vi "Prueba_comandos.vi"() -> ()   [LabVIEW 2010]
uses:
  <vilib>/Instr/_visa.llb/VISA Configure Serial Port (Instr).vi
panel:
  out "Comando leido":string
  in  "Leer":bool
  in  "Comando a escribir":string="WTt1 000000000"
  in  "Escribir":bool
  in  "stop":bool
  out "Error":errorcluster={"status"=TRUE, "code"=-1073807343, "source"="Property Node (arg 1) in VISA Configure Serial Port (Instr).vi->Prueba_comandos.vi"}
  in  "Puerto USB":refnum<visa-resource-name>="COM22"
  # "Prueba de comandos"
  # "johny.jaramillo@udea.edu.co"
  # "daniel.estrada1@udea.edu.co"
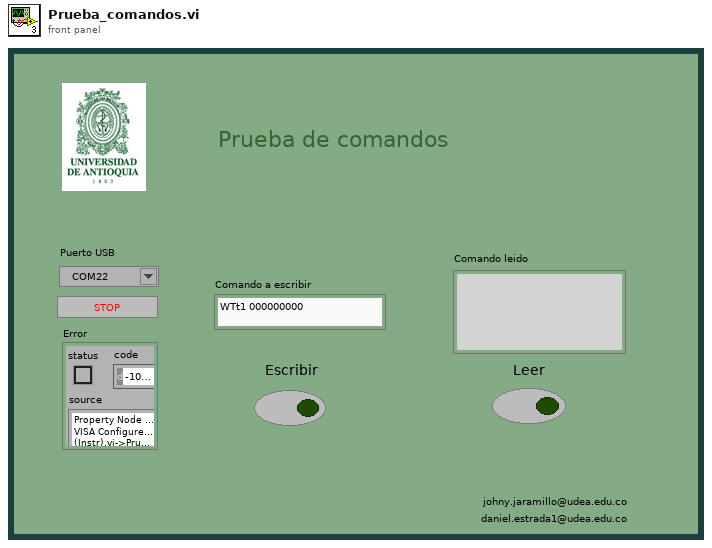
[diagram p1: front panel]
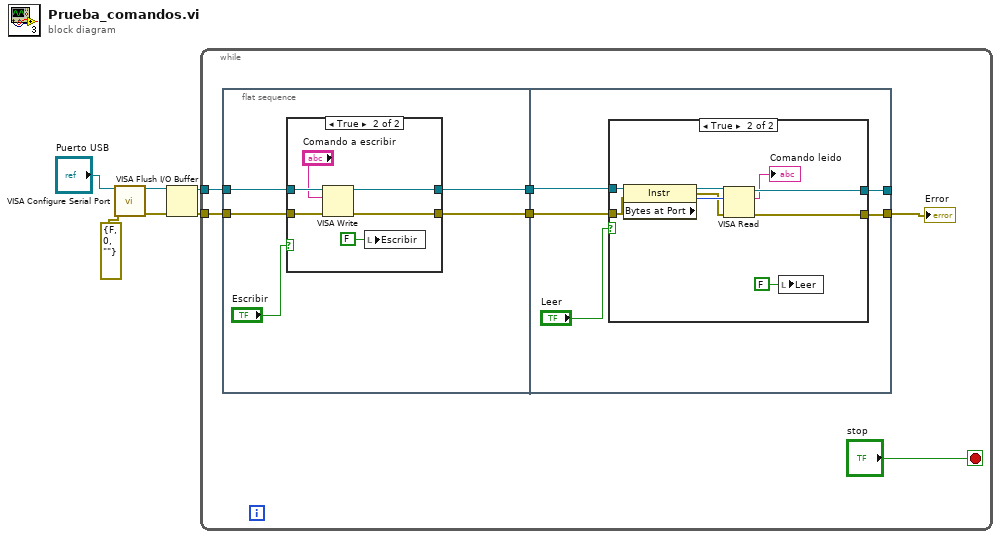
[diagram p0: block diagram]
diagram:
  n1 = call-poly "VISA Configure Serial Port"("VISA resource name"="Puerto USB", "error in (no error)"=errorcluster {"status"=FALSE, "code"=0, "source"=""}) -> ("VISA resource name out"=w4:refnum<visa-resource-name>, "error out"=w3:errorcluster)  [unwired: 12 in]
  n2 = VISA Flush I/O Buffer(VISA resource name=w4, error in (no error)=w3) -> (VISA resource name out=w2:refnum<visa-resource-name>, error out=w1:errorcluster)  [unwired: 1 in]
  n3 = while {
    tunnel: w2 -> [w10]
    tunnel: w1 -> [w9]
    stop <- "stop" stop-if-true
    n4 = flat-sequence {
      tunnel: [w15] -> w12
      tunnel: [w14] -> w11
      tunnel: w10 -> [w17]
      tunnel: w9 -> [w16]
      tunnel: w12 -> [w30]
      tunnel: w11 -> [w29]
      tunnel: [w28] -> _
      tunnel: [w27] -> w7
      frame #0 {
        n5 = case shown="True" "Escribir" {
          tunnel: w17 -> [w19 w25]
          tunnel: w16 -> [w18 w24]
          tunnel: [w19 w23] -> w15
          tunnel: [w18 w22] -> w14
          frame False {
          }
          frame True {
            n6 = VISA Write(VISA resource name=w25, write buffer="Comando a escribir", error in (no error)=w24) -> (VISA resource name out=w23:refnum<visa-resource-name>, error out=w22:errorcluster)  [unwired: 1 out]
            n7 = local write "Escribir"(FALSE ("Escribir")) -> ()
          }
        }
      }
      frame #1 {
        n8 = case shown="True" "Leer" {
          tunnel: w30 -> [w32 w39]
          tunnel: w29 -> [w31 w38]
          tunnel: [w32 w37] -> w28
          tunnel: [w31 w35] -> w27
          frame False {
          }
          frame True {
            n9 = property class="Instr"(reference=w39, error in=w38) -> (reference out=w41:refnum<visa-resource-name>, error out=w36:errorcluster, "Bytes at Port"=w40:u32)
            n10 = VISA Read(VISA resource name=w41, byte count=w40, error in (no error)=w36) -> (VISA resource name out=w37:refnum<visa-resource-name>, read buffer=→"Comando leido":string, error out=w35:errorcluster)  [unwired: 1 out]
            n11 = local write "Leer"(FALSE ("Leer")) -> ()
          }
        }
      }
    }
    "Error" <- w7
  }
